vi "U16 Array TO SGL Array.vi"(11 "REG U16":u16[](array[numeric])) -> (3 "SGL":sgl[](array[numeric]))   [LabVIEW 2019, in "Modbus DataType Conversation.lvlib"]
uses:
  Modbus DataType Conversation.lvlib
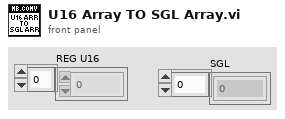
[diagram p1: front panel]
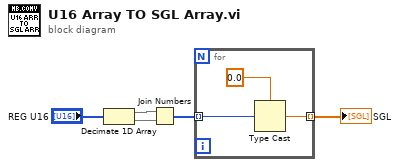
[diagram p0: block diagram]
diagram:
  n1 = Decimate 1D Array("REG U16") -> (w4:u16[], w3:u16[])
  n2 = Join Numbers(hi=w4, lo=w3) -> ((hi.lo)=w2:u32[])
  n3 = for {
    tunnel: w2 -> [w7] mode=indexing
    tunnel: [w6] -> w1 mode=indexing
    n4 = Type Cast(type=sgl 0.0, x=w7) -> (*(type *) &x=w6:sgl)
  }
  "SGL" <- w1
